vi "getStatus_action.vi"(0 "HGF_ImaqDx":refnum<class "HGF_ImaqDx.lvclass">, 5 "error in (no error)":errorcluster) -> (13 "Lost Counter":T1, 14 "dup HGF_ImaqDx":refnum<class "HGF_ImaqDx.lvclass">, 15 "Acquiring?":bool, 16 "Last Valid Buffer Index":u32, 17 "Last Valid Buffer Number":u32, 19 "error out":errorcluster)   [LabVIEW 2014, in "HGF_IMAQ.lvlib" / "HGF_ImaqDx.lvclass"]
doc: "Returns status information about the acquisition, such as the state of the acquisition and the last valid buffer acquired."
uses:
  HGF_ImaqDx.lvclass
  <resource>/objmgr/imaqdx.rc
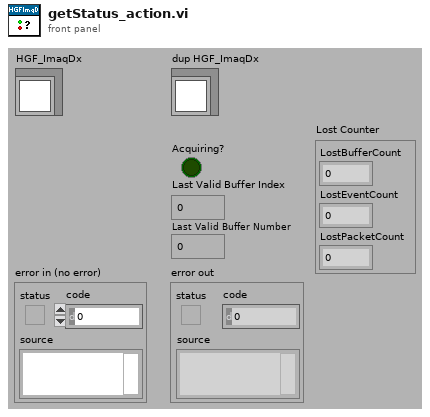
[diagram p1: front panel]
types:
  T1 = cluster{"LostBufferCount":u32, "LostEventCount":u32, "LostPacketCount":u32}
  T2 = typedef "IMAQdx.ctl" = refnum<k21>
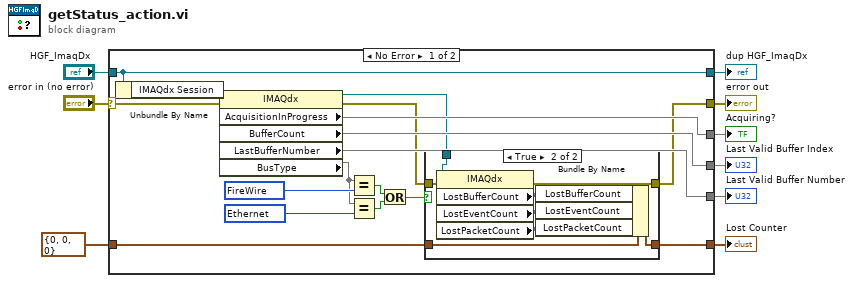
[diagram p0: block diagram]
diagram:
  n1 = case shown="No Error" "error in (no error)" {
    selector: "error in (no error)" -> [w23 w38]
    tunnel: "HGF_ImaqDx" -> [w24 w39]
    tunnel: [w25 _] -> w8
    tunnel: [w19 _] -> w7
    tunnel: [w20 _] -> w6
    tunnel: [w10 w38] -> w5
    tunnel: [w24 w39] -> w4
    tunnel: [w22 w37] -> w2
    tunnel: T1 {"LostBufferCount"=0, "LostEventCount"=0, "LostPacketCount"=0} ("Lost") -> [w21 w37]
    frame No Error {
      w16 = u32 825440564 items=["FireWire"=825440564, "Ethernet"=1768977972] ("BusType")
      w14 = u32 1768977972 items=["FireWire"=825440564, "Ethernet"=1768977972] ("BusType")
      n2 = Unbundle By Name(w24) -> ("IMAQdx Session"=w26:T2)
      n3 = property class="IMAQdx"(reference=w26, error in=w23) -> (reference out=w18:T2, error out=w17:errorcluster, "AcquisitionInProgress"=w25, "BufferCount"=w19, "LastBufferNumber"=w20, "BusType"=w15)
      n4 = Equal?(x=w15, y=w16) -> (x = y?=w13:bool)
      n5 = Equal?(x=w15, y=w14) -> (x = y?=w12:bool)
      n6 = Or(x=w13, y=w12) -> (x .or. y?=w11:bool)
      n7 = case shown="True" w11 {
        tunnel: [w28 w36] -> w22
        tunnel: w21 -> [w28 w35]
        tunnel: w18 -> [_ w34]
        tunnel: w17 -> [w27 w30]
        tunnel: [w27 w29] -> w10
        frame False {
        }
        frame True {
          n8 = property class="IMAQdx"(reference=w34, error in=w30) -> (error out=w29:errorcluster, "LostBufferCount"=w33, "LostEventCount"=w32, "LostPacketCount"=w31)  [unwired: 1 out]
          n9 = Bundle By Name(cluster=w35, "LostBufferCount"=w33, "LostEventCount"=w32, "LostPacketCount"=w31) -> (w36:T1)
        }
      }
    }
    frame Error {
    }
  }
  "error out" <- w5
  "dup HGF_ImaqDx" <- w4
  "Acquiring?" <- w8
  "Last Valid Buffer Index" <- w7
  "Last Valid Buffer Number" <- w6
  "Lost Counter" <- w2
